vi "dfd_Super Narrowband Filter Design Create Filter Array from Old Filter.vi"(8 "error in (no error)":errorcluster, 9 "error":i32, 11 "IFIR Coefficients":T2 {"Image Suppressor" format="%0.2e"; "Model Filter" format="%0.2e"}) -> (0 "error out":errorcluster, 2 "new filter type":T1(ring), 3 "multirate filters out":T3[](array[typedef]) {"mMRate_SumWl" min=1 max=32 step=1; "mMRate_InputIwl" min=1 max=32 step=1; "mMRate_GainWl" min=1 max=32 step=1; "mMRate_OutputWl" min=1 max=32 step=1; "mMRate_InputWl" min=1 max=32 step=1; "mMRate_CoefWl" min=1 max=32 step=1; "mMRate_Mode" items=["Default"=-1, "No Rate Change"=0, "Interpolation"=1, "Decimation"=2, "Interpolated"=3, "Rational"=4]})   [LabVIEW 2017, in "NI_DigFilter_Process.lvlib"]
doc: "Generates a set of filter coefficients to implement a digital interpolated FIR (IFIR) filter."
uses:
  <vilib>/addons/Digital Filter Design/NI_DigFilter_Process.lvlib
  <vilib>/addons/Digital Filter Design/_Objects.llb/DFD Multirate Filter Obj.ctl
  <vilib>/addons/Digital Filter Design/_Objects.llb/DFD Multirate Mode.ctl
  <vilib>/addons/Digital Filter Design/_Objects.llb/DFD Coef Norm Type.ctl
  <vilib>/addons/Digital Filter Design/_Objects.llb/DFD Round-off Mode.ctl
  <vilib>/addons/Digital Filter Design/_Objects.llb/DFD FXP MRate Multiply Mode.ctl
  <vilib>/addons/Digital Filter Design/_Misc.llb/dfd_Error Cluster From Error Code (Scalar).vi
  <vilib>/addons/Digital Filter Design/NI_DigFilterLicensed.lvlib
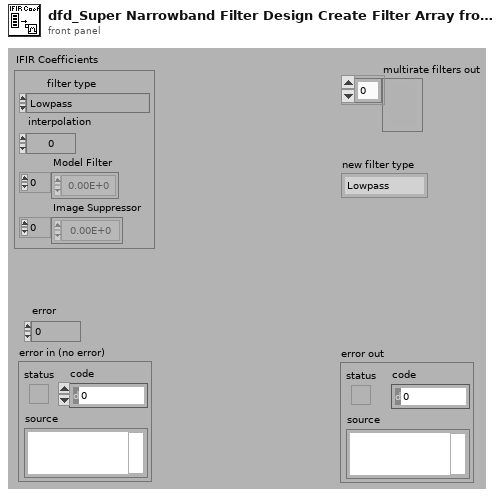
[diagram p1: front panel]
types:
  T1 = enum32{"Lowpass", "Highpass", "Bandpass", "Bandstop", "Wideband-Lowpass", "Wideband-Highpass"}
  T2 = cluster{"filter type":enum32{"Lowpass", "Highpass", "Bandpass", "Bandstop", "Wideband-Lowpass", "Wideband-Highpass"}, "interpolation":i32, "Model Filter":dbl[], "Image Suppressor":dbl[]}
  T3 = typedef "NI_DigFilterLicensed.lvlib/DFD Multirate Filter Obj.ctl" = cluster{"mMRate_Structure":enum16{"CIC", "FIR", "IIR", "Lattice"}, "mMRate_Mode":T4, "mMRate_Factor":i32, "mMRate_FIRParams":cluster{"mMRate_FIR_H":dbl[], "mMRate_FIR_IsNyquist?":bool, "mMRate_FIR_IsSymmetric?":bool}, "mMRate_CICParams":cluster{"mMRate_CIC_#Stage":i32, "mMRate_CIC_Lag":i32, "mMRate_CIC_Type":enum16{"Lowpass", "Highpass"}}, "mMRate_Order":i32, "mMRate_Version":string, "mMRate_Comments":string, "mMRate_RationalFactor":cluster{"mMRate_L":i32, "mMRate_M":i32}, "mMRate_Fs":dbl, "mMRate_Quantized?":bool, "mMRate_QFilterGain":dbl, "mMRate_CoefWl":i16, "mMRate_Scaling":cluster{"mMRate_ScaleByPowerOf2?":bool, "mMRate_ScaleType":T5}, "mMRate_InputWl":i16, "mMRate_OutputWl":i16, "mMRate_OutputMode":T6, "mMRate_MultMode":T7, "mMRate_BitPruning":bool, "mMRate_GainWl":i16, "mMRate_OutputFwl":i16, "mMRate_SumIwl":i16, "mMRate_InputIwl ":i16, "mMRate_SumWl":i16, "mMRate_CoefIwl":i16}
  T4 = typedef "NI_DigFilterLicensed.lvlib/DFD Multirate Mode.ctl" = i16
  T5 = typedef "NI_DigFilterLicensed.lvlib/DFD Coef Norm Type.ctl" = enum16{"No Norm", "Time Domain 1-Norm", "Time Domain 2-Norm", "Time Domain Inf-Norm"}
  T6 = typedef "NI_DigFilterLicensed.lvlib/DFD Round-off Mode.ctl" = enum16{"Nearest", "Truncation"}
  T7 = typedef "NI_DigFilterLicensed.lvlib/DFD FXP MRate Multiply Mode.ctl" = enum16{"Truncated", "Full"}
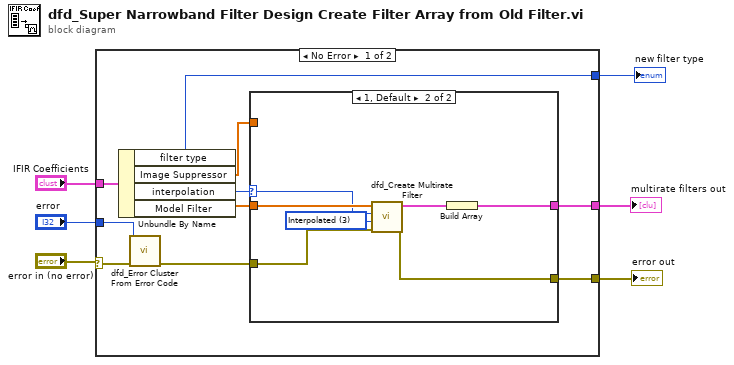
[diagram p0: block diagram]
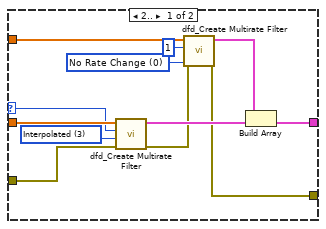
[diagram p2: hidden frame]
diagram:
  n1 = case shown="No Error" "error in (no error)" {
    selector: "error in (no error)" -> [w11 w36]
    tunnel: [w16 w36] -> w6
    tunnel: "IFIR Coefficients" -> [w15 _]
    tunnel: "error" -> [w13 _]
    tunnel: [w10 _] -> w2
    tunnel: [w7 _] -> w1
    frame No Error {
      n2 = Unbundle By Name(w15) -> ("filter type"=w10:T1, "Image Suppressor"=w14:dbl[], "interpolation"=w8:i32, "Model Filter"=w9:dbl[])
      n3 = call-poly <vilib>:"dfd_Error Cluster From Error Code.vi"("error in (no error)"=w11, "error code (0)"=w13) -> ("error out"=w12:errorcluster)  [unwired: 9 out]
      n4 = case shown="1, Default" w8 {
        selector: w8 -> [w27 w32]
        tunnel: [w20 w30] -> w16
        tunnel: w9 -> [w28 w35]
        tunnel: w14 -> [w24 _]
        tunnel: w12 -> [w25 w34]
        tunnel: [w19 w31] -> w7
        frame 2.. {
          w17 = T4 3 items=["Default"=-1, "No Rate Change"=0, "Interpolation"=1, "Decimation"=2, "Interpolated"=3] ("mode")
          w18 = T4 0 items=["Default"=-1, "No Rate Change"=0, "Interpolation"=1, "Decimation"=2, "Interpolated"=3] ("mode")
          n5 = call <vilib>:"dfd_Create Multirate Filter.vi"("error in (no error)"=w25, "mode"=w17, "factor"=w27, "h (n)"=w28) -> ("error out"=w21:errorcluster, "multirate filter out"=w26:T3)  [unwired: 1 in, 5 out]
          n6 = call <vilib>:"dfd_Create Multirate Filter.vi"("error in (no error)"=w21, "mode"=w18, "factor"=1, "h (n)"=w24) -> ("error out"=w20:errorcluster, "multirate filter out"=w22:T3)  [unwired: 1 in, 5 out]
          n7 = Build Array(w22, w26) -> (w19:T3[])
        }
        frame 1, Default {
          w29 = T4 3 items=["Default"=-1, "No Rate Change"=0, "Interpolation"=1, "Decimation"=2, "Interpolated"=3] ("mode")
          n8 = call <vilib>:"dfd_Create Multirate Filter.vi"("error in (no error)"=w34, "mode"=w29, "factor"=w32, "h (n)"=w35) -> ("error out"=w30:errorcluster, "multirate filter out"=w33:T3)  [unwired: 1 in, 5 out]
          n9 = Build Array(w33) -> (w31:T3[])
        }
      }
    }
    frame Error {
    }
  }
  "error out" <- w6
  "multirate filters out" <- w1
  "new filter type" <- w2
